vi "ScanOperationalMode.vi"(11 "operationalMode in":string) -> (3 "operationalMode out":T1)   [LabVIEW 2019, in "Universal Robot.lvclass"]
uses:
  Universal Robot.lvclass
  OperationalMode.ctl
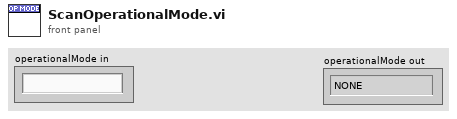
[diagram p1: front panel]
types:
  T1 = typedef "Universal Robot.lvclass/OperationalMode.ctl" = enum16{"NONE", "MANUAL", "AUTOMATIC"}
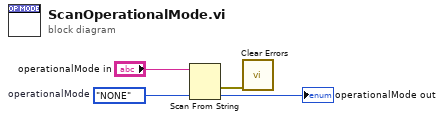
[diagram p0: block diagram]
diagram:
  w3 = OperationalMode."NONE"  # operationalMode
  n1 = Scan From String(input string="operationalMode in", default 1=w3) -> (error out=w1:errorcluster, output 1=→"operationalMode out":T1)  [unwired: 3 in, 2 out]
  n2 = call <vilib>:"Clear Errors.vi"("error in (no error)"=w1) -> ()  [unwired: 5 in, 2 out]
